vi "Proto Parser.vi"(8 "error in (no error)":errorcluster, 11 ".proto file path":path=path "C:/dev/labview-grpc-server/tests/data_marshal/data_marshal.proto") -> (0 "error out":errorcluster, 1 "gRPC Method Parameters":T4[](array[typedef]), 2 "gRPC Messages Parameters":T1[](array[typedef]))   [LabVIEW 2019, in "gRPC Scripting Tools.lvlib"]
uses:
  gRPC Scripting Tools.lvlib
  TypeDefs/RPC Method Parameters.ctl
  TypeDefs/Message Metadata (Scripting).ctl
  TypeDefs/Message Element Metadata (Scripting).ctl
  TypeDefs/Message Element Type.ctl
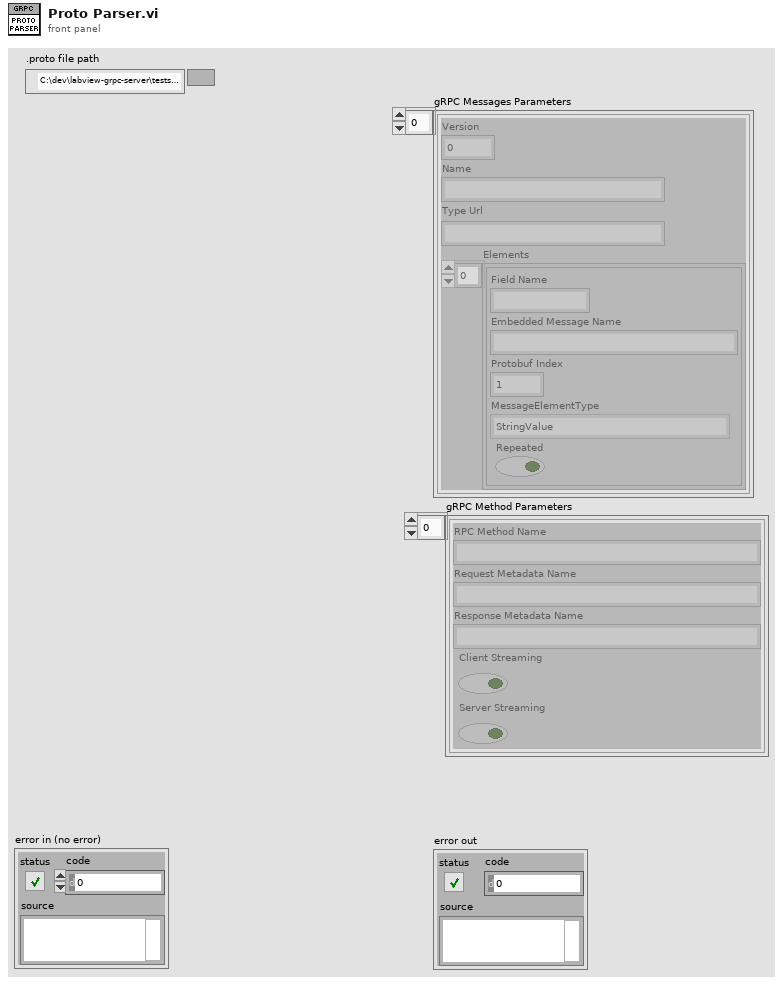
[diagram p1: front panel]
types:
  T1 = typedef "gRPC Scripting Tools.lvlib/Message Metadata (Scripting).ctl" = cluster{"Version":i32, "Name":string, "Type Url":string, "Elements":T2[]}
  T2 = typedef "gRPC Scripting Tools.lvlib/Message Element Metadata (Scripting).ctl" = cluster{"Field Name":string, "Embedded Message Name":string, "Protobuf Index":i32, "MessageElementType":T3, "Repeated":bool}
  T3 = typedef "gRPC Scripting Tools.lvlib/Message Element Type.ctl" = enum32{"Int32Value", "FloatValue", "DoubleValue", "BoolValue", "StringValue", "MessageValue", "Int64Value", "UInt32Value", "UInt64Value", "EnumValue", "Bytes", "Fixed64", "Fixed32", "SFixed64", "SFixed32", "SInt64", "SInt32"}
  T4 = typedef "gRPC Scripting Tools.lvlib/RPC Method Parameters.ctl" = cluster{"RPC Method Name":string, "Request Metadata Name":string, "Response Metadata Name":string, "Client Streaming":bool, "Server Streaming":bool}
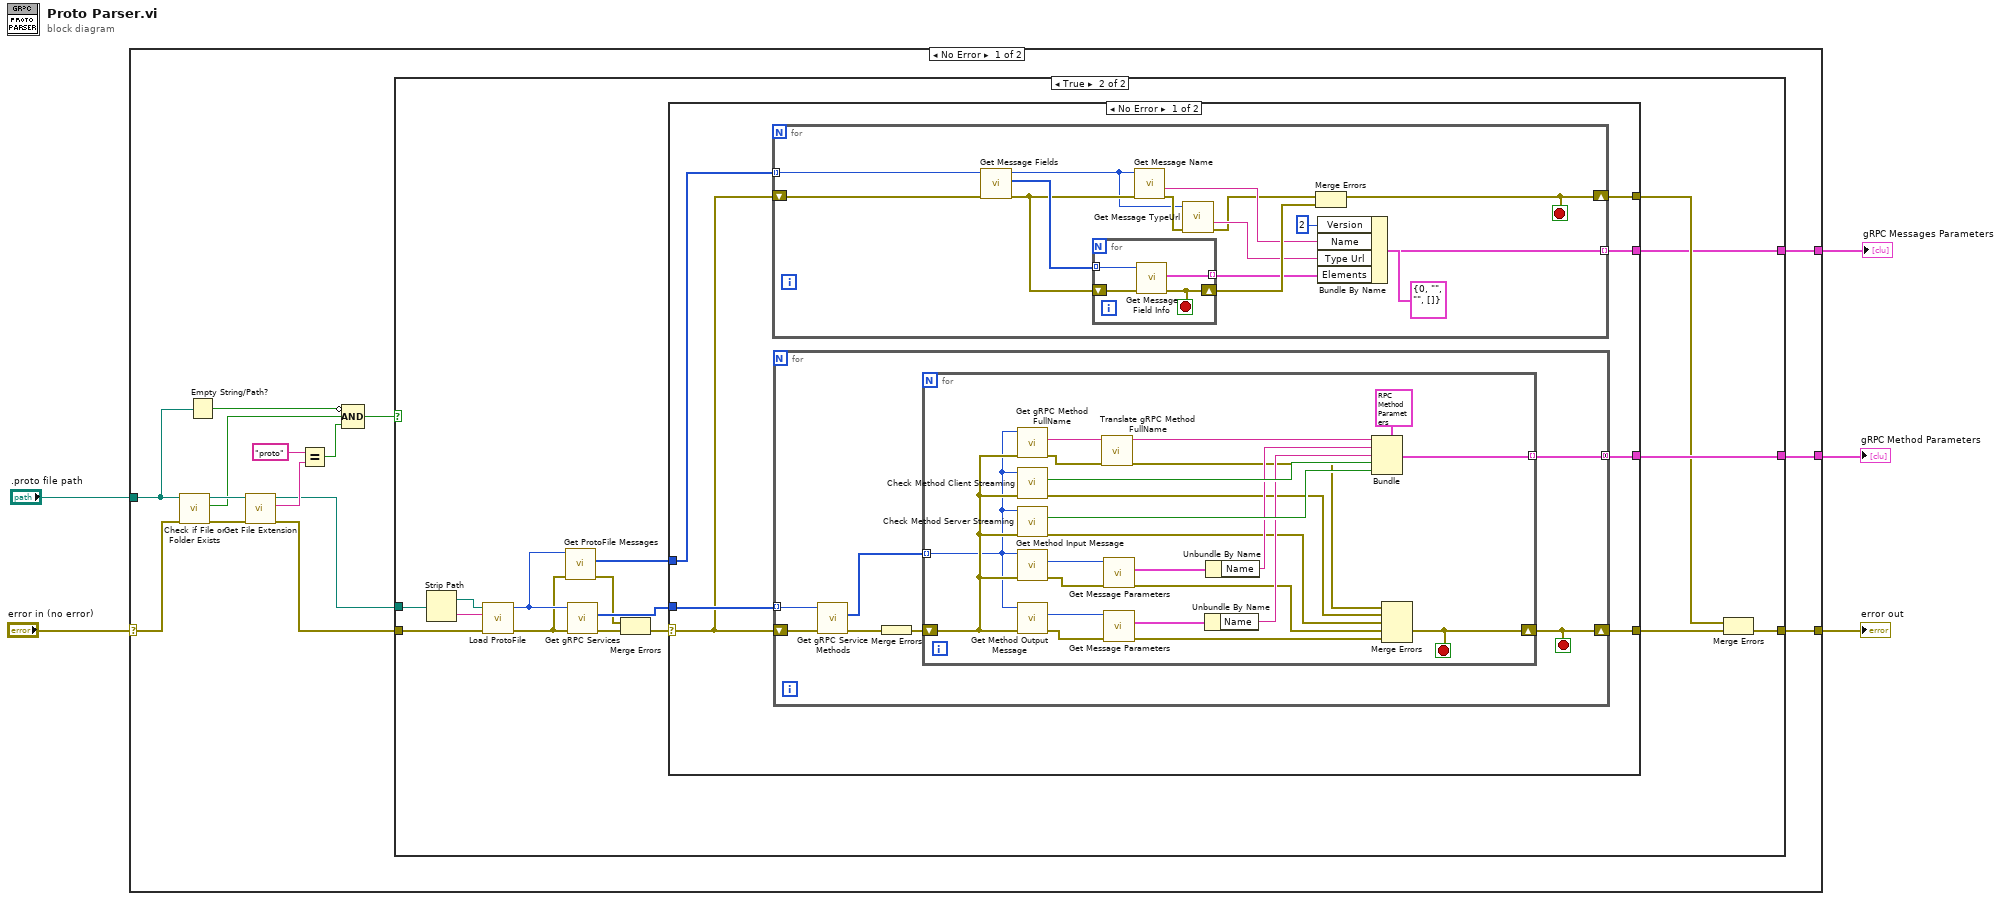
[diagram p0: block diagram]
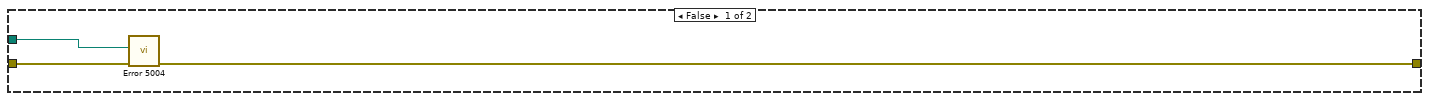
[diagram p2: hidden frame]
diagram:
  n1 = case shown="No Error" "error in (no error)" {
    selector: "error in (no error)" -> [w17 w97]
    tunnel: ".proto file path" -> [w18 _]
    tunnel: [w20 _] -> w5
    tunnel: [w19 w97] -> w4
    tunnel: [w6 _] -> w1
    frame No Error {
      n2 = call <vilib>:"Check if File or Folder Exists.vi"("error in (no error)"=w17, "path"=w18) -> ("error out"=w16:errorcluster, "file or folder exists?"=w11:bool, "dup path"=w15:path)  [unwired: 7 in]
      n3 = Empty String/Path?(string/path=w18) -> (empty?=w10:bool)
      n4 = call <vilib>:"Get File Extension.vi"("error in (no error)"=w16, "file"=w15) -> ("error out"=w7:errorcluster, "lowercase file extension"=w14:string, "dup file"=w8:path)  [unwired: 5 in, 2 out]
      n5 = Equal?(x="proto", y=w14) -> (x = y?=w12:bool)
      n6 = Compound Arithmetic op=AND(invert w10, w11, w12) -> (w9:bool)
      n7 = case shown="True" w9 {
        tunnel: [_ w36] -> w20
        tunnel: [w22 w25] -> w19
        tunnel: w8 -> [w21 w35]
        tunnel: w7 -> [w23 w34]
        tunnel: [_ w24] -> w6
        frame False {
          n8 = call "Error 5004.vi"("error in (no error)"=w23, "Proto file path"=w21) -> ("error out"=w22:errorcluster)  [unwired: 9 in]
        }
        frame True {
          n9 = Strip Path(path=w35) -> (stripped path=w39:path, name=w38:string)
          n10 = call "Load ProtoFile.vi"("error in (no error)"=w34, "File Name"=w38, "File Base path"=w39) -> ("error out"=w31:errorcluster, "protoFile ref out"=w32:u64)  [unwired: 7 in]
          n11 = call "Get ProtoFile Messages.vi"("error in (no error)"=w31, "Protofile ref in"=w32) -> ("error out"=w30:errorcluster, "ProtoFile Messages"=w28:u64[])  [unwired: 7 in, 1 out]
          n12 = call "Get gRPC Services.vi"("error in (no error)"=w31, "protoFile ref in"=w32) -> ("error out"=w33:errorcluster, "services"=w37:u64[])  [unwired: 7 in, 1 out]
          n13 = Merge Errors(w30, w33) -> (w29:errorcluster)
          n14 = case shown="No Error" w29 {
            selector: w29 -> [w42 w96]
            tunnel: w37 -> [w46 _]
            tunnel: [w45 _] -> w36
            tunnel: [w44 w96] -> w27
            tunnel: w28 -> [w43 _]
            tunnel: [w41 _] -> w26
            tunnel: [w40 _] -> w24
            frame No Error {
              n15 = for {
                tunnel: w43 -> [w61] mode=indexing
                shift-right: [w54] -> w41
                shift-left: w42 -> [w58]
                tunnel: [w55] -> w40 mode=indexing
                stop <- w54 stop-if-true
                n16 = call "Get Message Fields.vi"("error in (no error)"=w58, "Message ref in"=w61) -> ("error out"=w57:errorcluster, "Field refs"=w60:u64[], "Message ref out"=w50:u64)  [unwired: 7 in]
                n17 = for {
                  tunnel: w60 -> [w65] mode=indexing
                  tunnel: [w64] -> w52 mode=indexing
                  shift-right: [w62] -> w56
                  shift-left: w57 -> [w63]
                  stop <- w62 stop-if-true
                  n18 = call "Get Message Field Info.vi"("error in (no error)"=w63, "Message Field ref in"=w65) -> ("error out"=w62:errorcluster, "Field Info"=w64:T2)  [unwired: 7 in, 1 out]
                }
                n19 = call "Get Message Name.vi"("error in (no error)"=w57, "Message ref in"=w50) -> ("error out"=w51:errorcluster, "Message Name"=w53:string)  [unwired: 7 in, 1 out]
                n20 = call "Get Message TypeUrl.vi"("error in (no error)"=w51, "Message ref in"=w50) -> ("error out"=w48:errorcluster, "Message Name"=w49:string)  [unwired: 7 in, 1 out]
                n21 = Merge Errors(w48, w56) -> (w54:errorcluster)
                n22 = Bundle By Name(cluster=T1 {"Version"=0, "Name"="", "Type Url"="", "Elements"=[]} ("Message Metadata"), "Version"=2, "Name"=w53, "Type Url"=w49, "Elements"=w52) -> (w55:T1)
              }
              n23 = for {
                tunnel: w46 -> [w72] mode=indexing
                tunnel: [w71] -> w45 mode=concatenating
                shift-right: [w66] -> w44
                shift-left: w42 -> [w69]
                stop <- w66 stop-if-true
                n24 = call "Get gRPC Service Methods.vi"("error in (no error)"=w69, "Service ref in"=w72) -> ("error out"=w68:errorcluster, "Service Methods"=w70:u64[])  [unwired: 7 in, 1 out]
                n25 = Merge Errors(w68) -> (w67:errorcluster)
                n26 = for {
                  tunnel: w70 -> [w77] mode=indexing
                  tunnel: [w95] -> w71 mode=indexing
                  shift-right: [w79] -> w66
                  shift-left: w67 -> [w78]
                  stop <- w79 stop-if-true
                  n27 = call "Get gRPC Method FullName.vi"("error in (no error)"=w78, "Method ref in"=w77) -> ("error out"=w76:errorcluster, "Method Full Name"=w75:string)  [unwired: 7 in, 1 out]
                  n28 = call "Check Method Client Streaming.vi"("error in (no error)"=w78, "Method ref in"=w77) -> ("error out"=w83:errorcluster, "is Client Streaming"=w94:bool)  [unwired: 7 in, 1 out]
                  n29 = call "Check Method Server Streaming.vi"("error in (no error)"=w78, "Method ref in"=w77) -> ("error out"=w82:errorcluster, "is Server Streaming"=w93:bool)  [unwired: 7 in, 1 out]
                  n30 = call "Get Method Input Message.vi"("error in (no error)"=w78, "Method ref in"=w77) -> ("error out"=w88:errorcluster, "Message ref out"=w91:u64)  [unwired: 7 in, 1 out]
                  n31 = call "Get Method Output Message.vi"("error in (no error)"=w78, "Method ref in"=w77) -> ("error out"=w89:errorcluster, "Message ref out"=w90:u64)  [unwired: 7 in, 1 out]
                  n32 = call "Translate gRPC Method FullName.vi"("error in (no error)"=w76, "Method Full Name in"=w75) -> ("error out"=w73:errorcluster, "Method Full Name out"=w74:string)  [unwired: 8 in]
                  n33 = call "Get Message Parameters.vi"("error in (no error)"=w88, "Message ref in"=w91) -> ("error out"=w81:errorcluster, "Message Metadata"=w85:T1)  [unwired: 7 in, 1 out]
                  n34 = call "Get Message Parameters.vi"("error in (no error)"=w89, "Message ref in"=w90) -> ("error out"=w80:errorcluster, "Message Metadata"=w84:T1)  [unwired: 7 in, 1 out]
                  n35 = Unbundle By Name(w84) -> ("Name"=w86:string)
                  n36 = Unbundle By Name(w85) -> ("Name"=w87:string)
                  n37 = Bundle(cluster=T4 {"RPC Method Name"="/queryserver.QueryServer/Invoke", "Request Metadata Name"="InvokeRequest", "Response Metadata Name"="InvokeResponse", "Client Streaming"=FALSE, "Server Streaming"=FALSE}, "RPC Method Name"=w74, "Request Metadata Name"=w87, "Response Metadata Name"=w86, "Client Streaming"=w94, "Server Streaming"=w93) -> (w95:T4)
                  n38 = Merge Errors(w73, w83, w82, w81, w80) -> (w79:errorcluster)
                }
              }
            }
            frame Error {
            }
          }
          n39 = Merge Errors(w26, w27) -> (w25:errorcluster)
        }
      }
    }
    frame Error {
    }
  }
  "gRPC Method Parameters" <- w5
  "error out" <- w4
  "gRPC Messages Parameters" <- w1
